vi "Vision Align.vi"(10 "Dashboard Drivetrain Command":T2 {"Vision PID gains"."derivative time (Td, min)" format="%.3f"; "Vision PID gains"."integral time (Ti, min)" format="%.3f"; "Vision PID gains"."proportional gain (Kc)" format="%.3f"}, 11 "Goal Vision Packet":T1) -> (2 "Aligned?":bool, 3 "Turn Power":dbl)   [LabVIEW 2015]
uses:
  Common Code/Dashboard Drivetrain Command.ctl
  Common Code/Drivetrain Vision.ctl
  Common Code/Goal Vision Packet.ctl
  <vilib>/addons/control/pid/pid.llb/PID (DBL).vi
  <vilib>/addons/control/pid/NI_PID_pid.lvlib
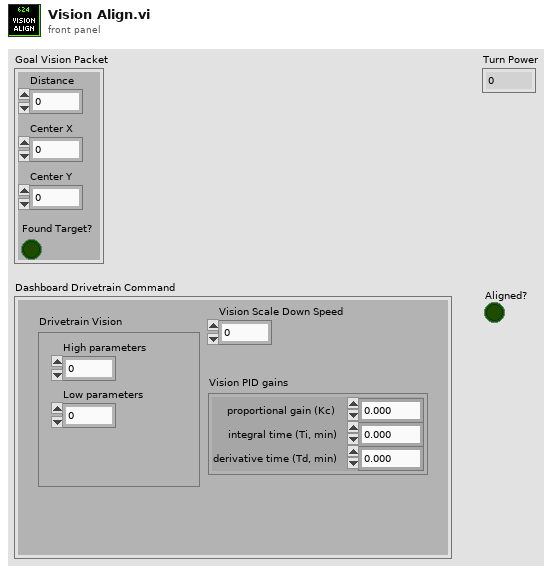
[diagram p1: front panel]
types:
  T1 = typedef "Goal Vision Packet.ctl" = cluster{"Distance":dbl, "Center X":dbl, "Center Y":dbl, "Found Target?":bool}
  T2 = typedef "Dashboard Drivetrain Command.ctl" = cluster{"Drivetrain Vision":T3, "Vision Scale Down Speed":dbl, "Vision PID gains":cluster{"proportional gain (Kc)":dbl, "integral time (Ti, min)":dbl, "derivative time (Td, min)":dbl}}
  T3 = typedef "Drivetrain Vision.ctl" = cluster{"High parameters":dbl, "Low parameters":dbl}
  T4 = cluster{"proportional gain (Kc)":dbl, "integral time (Ti, min)":dbl, "derivative time (Td, min)":dbl}
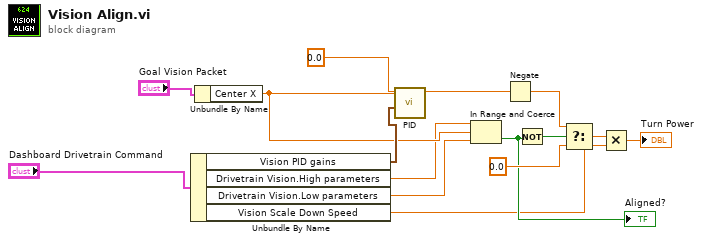
[diagram p0: block diagram]
diagram:
  n1 = Unbundle By Name("Dashboard Drivetrain Command") -> ("Vision PID gains"=w13:T4, "Drivetrain Vision.High parameters"=w3:dbl, "Drivetrain Vision.Low parameters"=w4:dbl, "Vision Scale Down Speed"=w9:dbl)
  n2 = Unbundle By Name("Goal Vision Packet") -> ("Center X"=w8:dbl)
  n3 = call-poly <vilib>:"PID.vi"("PID gains"=w13, "process variable"=w8, "setpoint"=0.0) -> ("output"=w14:dbl)  [unwired: 7 in, 1 out]
  n4 = In Range and Coerce(upper limit=w3, x=w8, lower limit=w4) -> (In Range?=w10:bool)  [unwired: 1 out]
  "Aligned?" <- w10
  n5 = Negate(x=w14) -> (-x=w15:dbl)
  n6 = Not(x=w10) -> (.not. x?=w11:bool)
  n7 = Select(t=w15, s=w11, f=0.0 ("t")) -> (s? t:f=w5:dbl)
  n8 = Multiply(x=w5, y=w9) -> (x*y=→"Turn Power":dbl)
